vi "Request Update from Process.vi"(8 "error in (no error)":errorcluster, 11 "Ilde in":refnum<class "Ready.lvclass">) -> (0 "error out":errorcluster, 3 "Ilde out":refnum<class "Ready.lvclass">)   [LabVIEW 2014]
doc: "Sends the Update message to the Process Actor."
uses:
  Process State/CoordinatorState.lvclass
  labview/1512/State Pattern Actor Example/Process Actor/Process Messages/Update Msg/Update Msg.lvclass
  Ready.lvclass
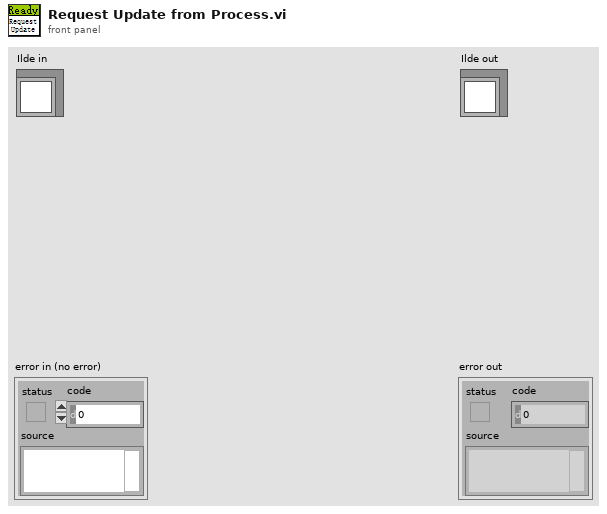
[diagram p1: front panel]
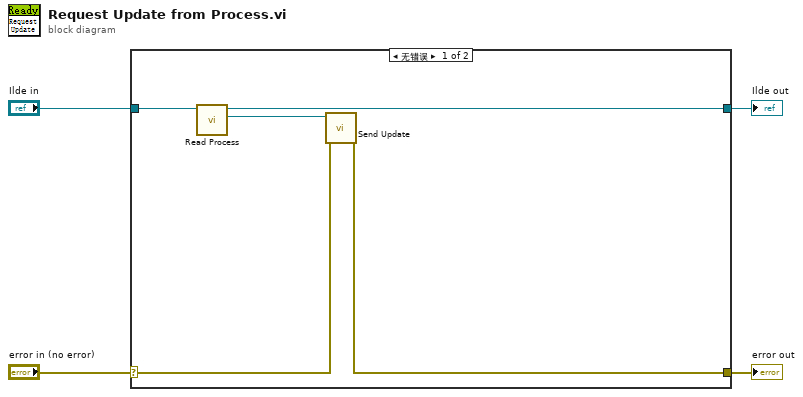
[diagram p0: block diagram]
diagram:
  n1 = case shown="无错误" "error in (no error)" {
    selector: "error in (no error)" -> [w6 w11]
    tunnel: [w5 w11] -> w3
    tunnel: [w8 w10] -> w1
    tunnel: "Ilde in" -> [w9 w10]
    frame No Error {
      n2 = call "Read Process.vi"("CommonState in"=w9) -> ("Process Enqueuer"=w7:refnum<class "Message Enqueuer.lvclass">, "CommonState out"=w8:refnum<class "Ready.lvclass">)  [unwired: 9 in]
      n3 = call "Send Update.vi"("error in (no error)"=w6, "Message Enqueuer"=w7) -> ("error out"=w5:errorcluster)  [unwired: 8 in, 1 out]
    }
    frame Error {
    }
  }
  "error out" <- w3
  "Ilde out" <- w1
